vi "Select Signals.vi"(8 "Error In":errorcluster, 10 "Selection":cluster{"Type":T2, "Index(es)":i32[]}[](xcontrol), 11 "DATA IN":T1) -> (0 "Error Out":errorcluster, 2 "Fs":u32, 3 "Array":waveform(dbl)[](array[waveform]))   [LabVIEW 2017, in "Signal Selector.lvlib"]
uses:
  Signal Selector.lvlib
  Selection Folder/Selection.xctl
  PMU Buffer/Buffer DATA OUT ordered.ctl
  <vilib>/Analysis/baseanly.llb/Mean (DBL).vi
  <vilib>/Analysis/NI_AALPro.lvlib
  <vilib>/Analysis/NI_AALBase.lvlib
  PMU Buffer/PMU data buffer.lvlib
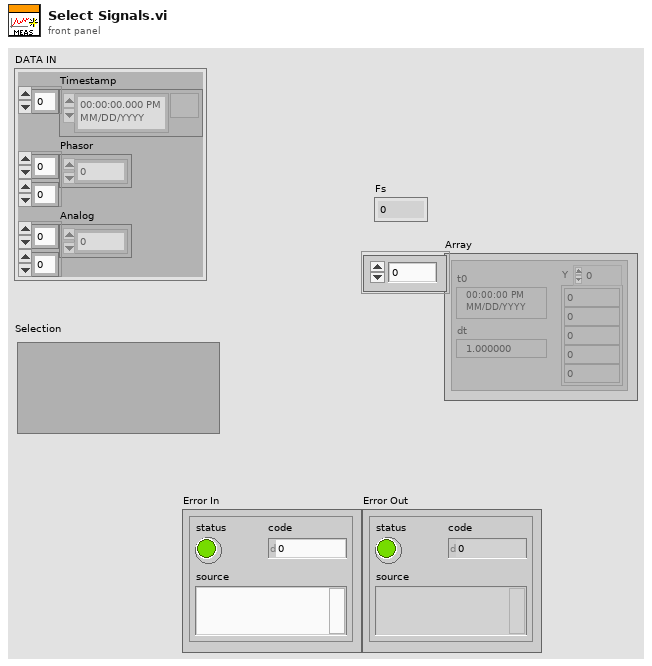
[diagram p1: front panel]
types:
  T1 = typedef "PMU data buffer.lvlib/Buffer DATA OUT ordered.ctl" = cluster{"Timestamp":timestamp[], "Phasor":csg[][], "Analog":sgl[][]}
  T2 = typedef "Selection.xctl/Signal types.ctl" = enum16{"Disable", "Frequency", "Phasor Mag", "Phasor Ang", "Angle Diff"}
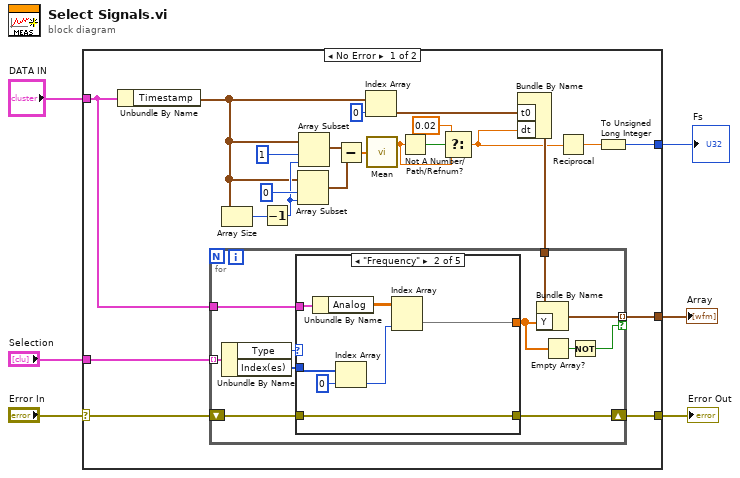
[diagram p0: block diagram]
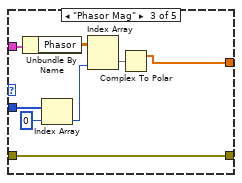
[diagram p3: hidden frame]
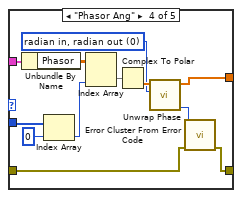
[diagram p4: hidden frame]
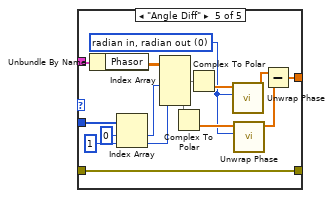
[diagram p5: hidden frame]
diagram:
  n1 = case shown="No Error" "Error In" {
    selector: "Error In" -> [w25 w84]
    tunnel: "Selection" -> [w28 _]
    tunnel: [w27 _] -> w6
    tunnel: [w24 w84] -> w4
    tunnel: [w15 _] -> w2
    tunnel: "DATA IN" -> [w14 _]
    frame No Error {
      n2 = Unbundle By Name(w14) -> ("Timestamp"=w11:timestamp[])
      n3 = Array Size(array=w11) -> (size(s)=w21:i32)
      n4 = Decrement(x=w21) -> (x-1=w20:i32)
      n5 = Array Subset(array=w11, index=0, length=w20) -> (w18:timestamp[])
      n6 = Array Subset(array=w11, index=1, length=w20) -> (w19:timestamp[])
      n7 = Subtract(x=w19, y=w18) -> (x-y=w17:dbl[])
      n8 = Index Array(array=w11, index=0) -> (element=w12:timestamp)
      n9 = call-poly <vilib>:"Mean.vi"("X"=w17) -> ("mean"=w9:dbl)  [unwired: 1 out]
      n10 = Not A Number/Path/Refnum?(number/path/refnum=w9) -> (NaN/Path/Refnum?=w10:bool)
      n11 = Select(t=0.02, s=w10, f=w9) -> (s? t:f=w7:dbl)
      n12 = Bundle By Name("t0"=w12, "dt"=w7) -> (w26:waveform(dbl))  [unwired: 1 in]
      n13 = for {
        tunnel: w28 -> [w39] mode=indexing
        tunnel: w14 -> [w36]
        tunnel: [w35] -> w27 mode=indexing if=w29
        tunnel: w26 -> [w34]
        shift-right: [w32] -> w24
        shift-left: w25 -> [w33]
        n14 = Unbundle By Name(w39) -> ("Type"=w38:T2, "Index(es)"=w37:i32[])
        n15 = case shown="\"Frequency\"" w38 {
          tunnel: w37 -> [_ w45 w50 w59 w72]
          tunnel: w36 -> [_ w46 w55 w67 w83]
          tunnel: [_ w41 w52 w62 w74] -> w31
          tunnel: w33 -> [w40 w47 w51 w56 w73]
          tunnel: [w40 w47 w51 w61 w73] -> w32
          frame "Disable", Default {
          }
          frame "Frequency" {
            n16 = Unbundle By Name(w46) -> ("Analog"=w43:sgl[][])
            n17 = Index Array(array=w45, index=0) -> (element=w42:i32)
            n18 = Index Array(array=w43, index (col)=w42) -> (element=w41:sgl[])  [unwired: 1 in]
          }
          frame "Phasor Mag" {
            n19 = Unbundle By Name(w55) -> ("Phasor"=w54:csg[][])
            n20 = Index Array(array=w50, index=0) -> (element=w48:i32)
            n21 = Index Array(array=w54, index (col)=w48) -> (element=w53:csg[])  [unwired: 1 in]
            n22 = Complex To Polar(r * e^(i*theta)=w53) -> (r=w52:sgl[])  [unwired: 1 out]
          }
          frame "Phasor Ang" {
            w63 = 0 items=["radian in, radian out", "radian in, degree out", "degree in, degree out", "degree in, radian out"] ("phase unit")
            n23 = Unbundle By Name(w67) -> ("Phasor"=w66:csg[][])
            n24 = Index Array(array=w59, index=0) -> (element=w58:i32)
            n25 = Index Array(array=w66, index (col)=w58) -> (element=w65:csg[])  [unwired: 1 in]
            n26 = Complex To Polar(r * e^(i*theta)=w65) -> (theta=w64:sgl[])  [unwired: 1 out]
            n27 = call <vilib>:"Unwrap Phase.vi"("phase unit"=w63, "Phase"=w64) -> ("error"=w60:i32, "Unwrapped Phase"=w62:dbl[])  [unwired: 8 in]
            n28 = call <vilib>:"Error Cluster From Error Code.vi"("error in (no error)"=w56, "error code (0)"=w60) -> ("error out"=w61:errorcluster)  [unwired: 7 in]
          }
          frame "Angle Diff" {
            w77 = 0 items=["radian in, radian out", "radian in, degree out", "degree in, degree out", "degree in, radian out"] ("phase unit")
            n29 = Unbundle By Name(w83) -> ("Phasor"=w82:csg[][])
            n30 = Index Array(array=w72, index #1=0 ("index"), index #2=1 ("index")) -> (element #1=w69:i32, element #2=w68:i32)
            n31 = Index Array(array=w82, index (col) #1=w69, index (col) #2=w68) -> (element #1=w81:csg[], element #2=w80:csg[])  [unwired: 2 in]
            n32 = Complex To Polar(r * e^(i*theta)=w80) -> (theta=w79:sgl[])  [unwired: 1 out]
            n33 = Complex To Polar(r * e^(i*theta)=w81) -> (theta=w78:sgl[])  [unwired: 1 out]
            n34 = call <vilib>:"Unwrap Phase.vi"("phase unit"=w77, "Phase"=w78) -> ("Unwrapped Phase"=w76:dbl[])  [unwired: 8 in, 1 out]
            n35 = call <vilib>:"Unwrap Phase.vi"("phase unit"=w77, "Phase"=w79) -> ("Unwrapped Phase"=w75:dbl[])  [unwired: 8 in, 1 out]
            n36 = Subtract(x=w76, y=w75) -> (x-y=w74:dbl[])
          }
        }
        n37 = Bundle By Name(cluster=w34, "Y"=w31) -> (w35:waveform(dbl))
        n38 = Empty Array?(array=w31) -> (empty?=w30:bool)
        n39 = Not(x=w30) -> (.not. x?=w29:bool)
      }
      n40 = Reciprocal(x=w7) -> (1/x=w16:dbl)
      n41 = To Unsigned Long Integer(number=w16) -> (unsigned 32bit integer=w15:u32)
    }
    frame Error {
    }
  }
  "Array" <- w6
  "Error Out" <- w4
  "Fs" <- w2
